vi "GameboardToNumeric.vi"(10 "CurrentPlayer":T1, 11 "Gameboard":T2) -> (3 "NumericGameboard":i8[](array[numeric]))   [LabVIEW 2020]
uses:
  controls/Gameboard Data.ctl
  controls/Player.ctl
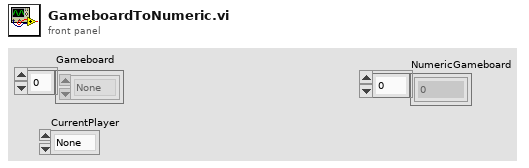
[diagram p1: front panel]
types:
  T1 = typedef "Player.ctl" = enum16{"None", "Player 1", "Player 2"}
  T2 = typedef "Gameboard Data.ctl" = enum16{"None", "Player 1", "Player 2"}[]
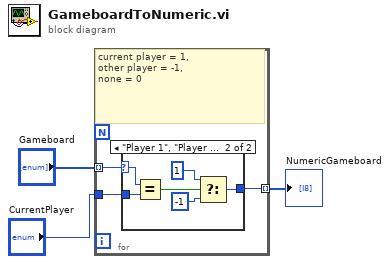
[diagram p0: block diagram]
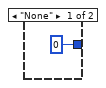
[diagram p2: hidden frame]
diagram:
  n1 = for {
    tunnel: "Gameboard" -> [w6] mode=indexing
    tunnel: "CurrentPlayer" -> [w5]
    tunnel: [w4] -> w1 mode=indexing
    # "current player = 1,\nother player = -1,\nnone = 0"
    n2 = case shown="\"Player 1\", \"Player 2\"" w6 {
      selector: w6 -> [_ w13]
      tunnel: w5 -> [_ w12]
      tunnel: [0 w8] -> w4
      frame "None" {
      }
      frame "Player 1", "Player 2" {
        n3 = Equal?(x=w13, y=w12) -> (x = y?=w11:bool)
        n4 = Select(t=1, s=w11, f=-1) -> (s? t:f=w8:i32)
      }
    }
  }
  "NumericGameboard" <- w1
